vi "ClsGetNextMultipleSamplesSingleChannelDevice.vi"(7 "Time out(ms)":i32, 8 "error in (no error)":errorcluster, 10 "Number of Samples":i32, 11 "Connection In":u32) -> (0 "error out":errorcluster, 1 "If Timeout?":bool, 2 "_Data":dbl[][](array[numeric]), 3 "Connection Out":u32)   [LabVIEW 2010]
doc: "Get Next Multiple Samples:\n\nThis function is used for single channel devices. This function is used to get the next multiple valid samples from device. Use this function to avoid the overheads for having to call Get Next Sample subVI once to read each sample. It is especially useful when the data rate is high. This function is block but with timeout input available.\n\nConnection In[Input]: the connection handle which is initially created by Open Connection subVI.\n\nTimeout(milisecond)[Input]: in miliseconds, the subvi will return after the timeout no matter enough data are read or not. If set to -1, the timeout will be infinity and it will block until enough data are read.\n\nNumber of Samples[Input]: the number of samples to read for each call. The maximum of this number is only determined by the available memory of your PC.\n\n\nData[Output]: The two dimensional array for data. Note that you can use Get Signal IDs subVI to see the ordering of signal IDs correspondent to this data array. The first dimension is for different samples and the second dimension is for different signals. The number of samples may be less than expected if timeout.\n\nTimeout?[Output]: Whether the return of the function is a result of timeout.\n\nConnection Out[Output]: the connection handle output which could be used for next subVI refering to the same connection."
uses:
  tmp/CHRocodile VIS 1.1/dependent dlls/CHRocodileDLL.dll
panel:
  out "Number of data points":i32
  out "Singal IDs":i32[](array[numeric])
  out "Number of signals":i32
  out "initialized array":dbl[][](array[numeric])
  out "sucessful size check?":i32
  out "number of loops with check":i32
  out "Nr of Samples Returned":i32
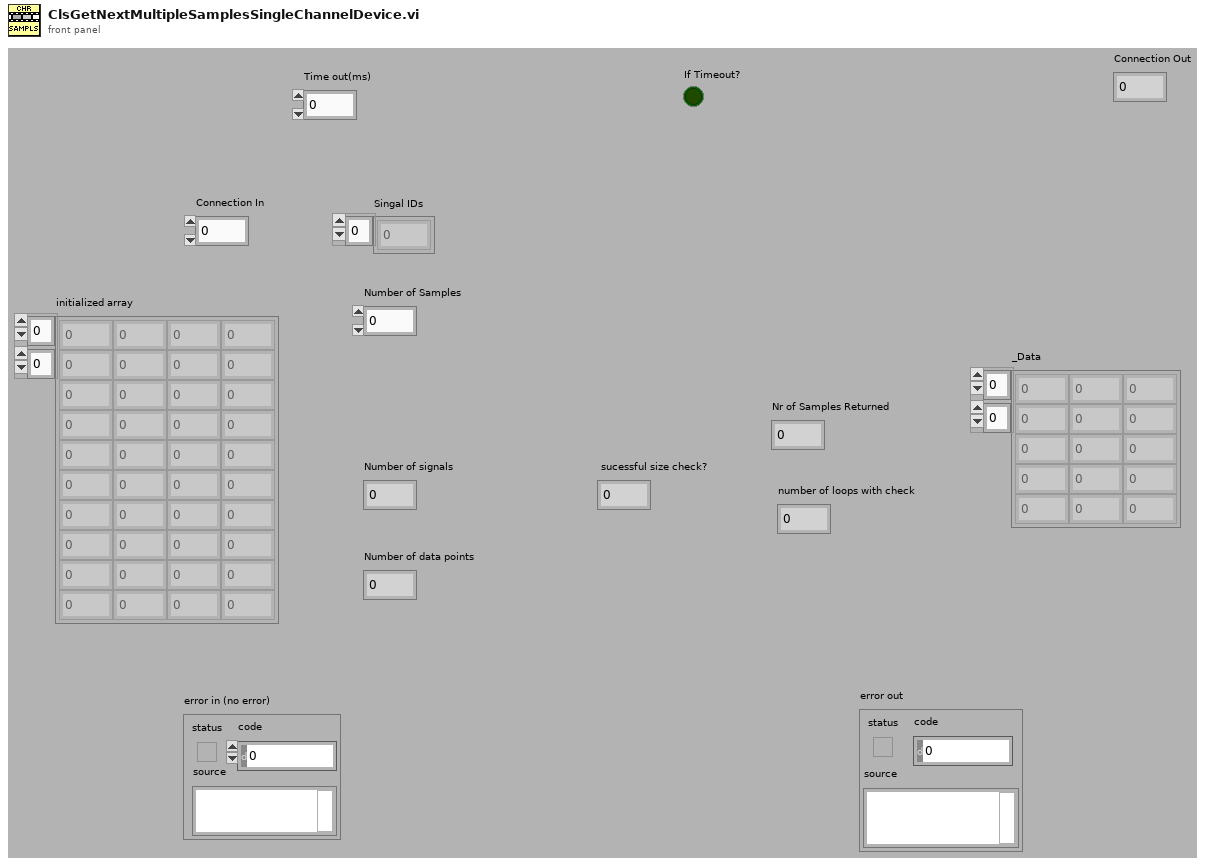
[diagram p1: front panel]
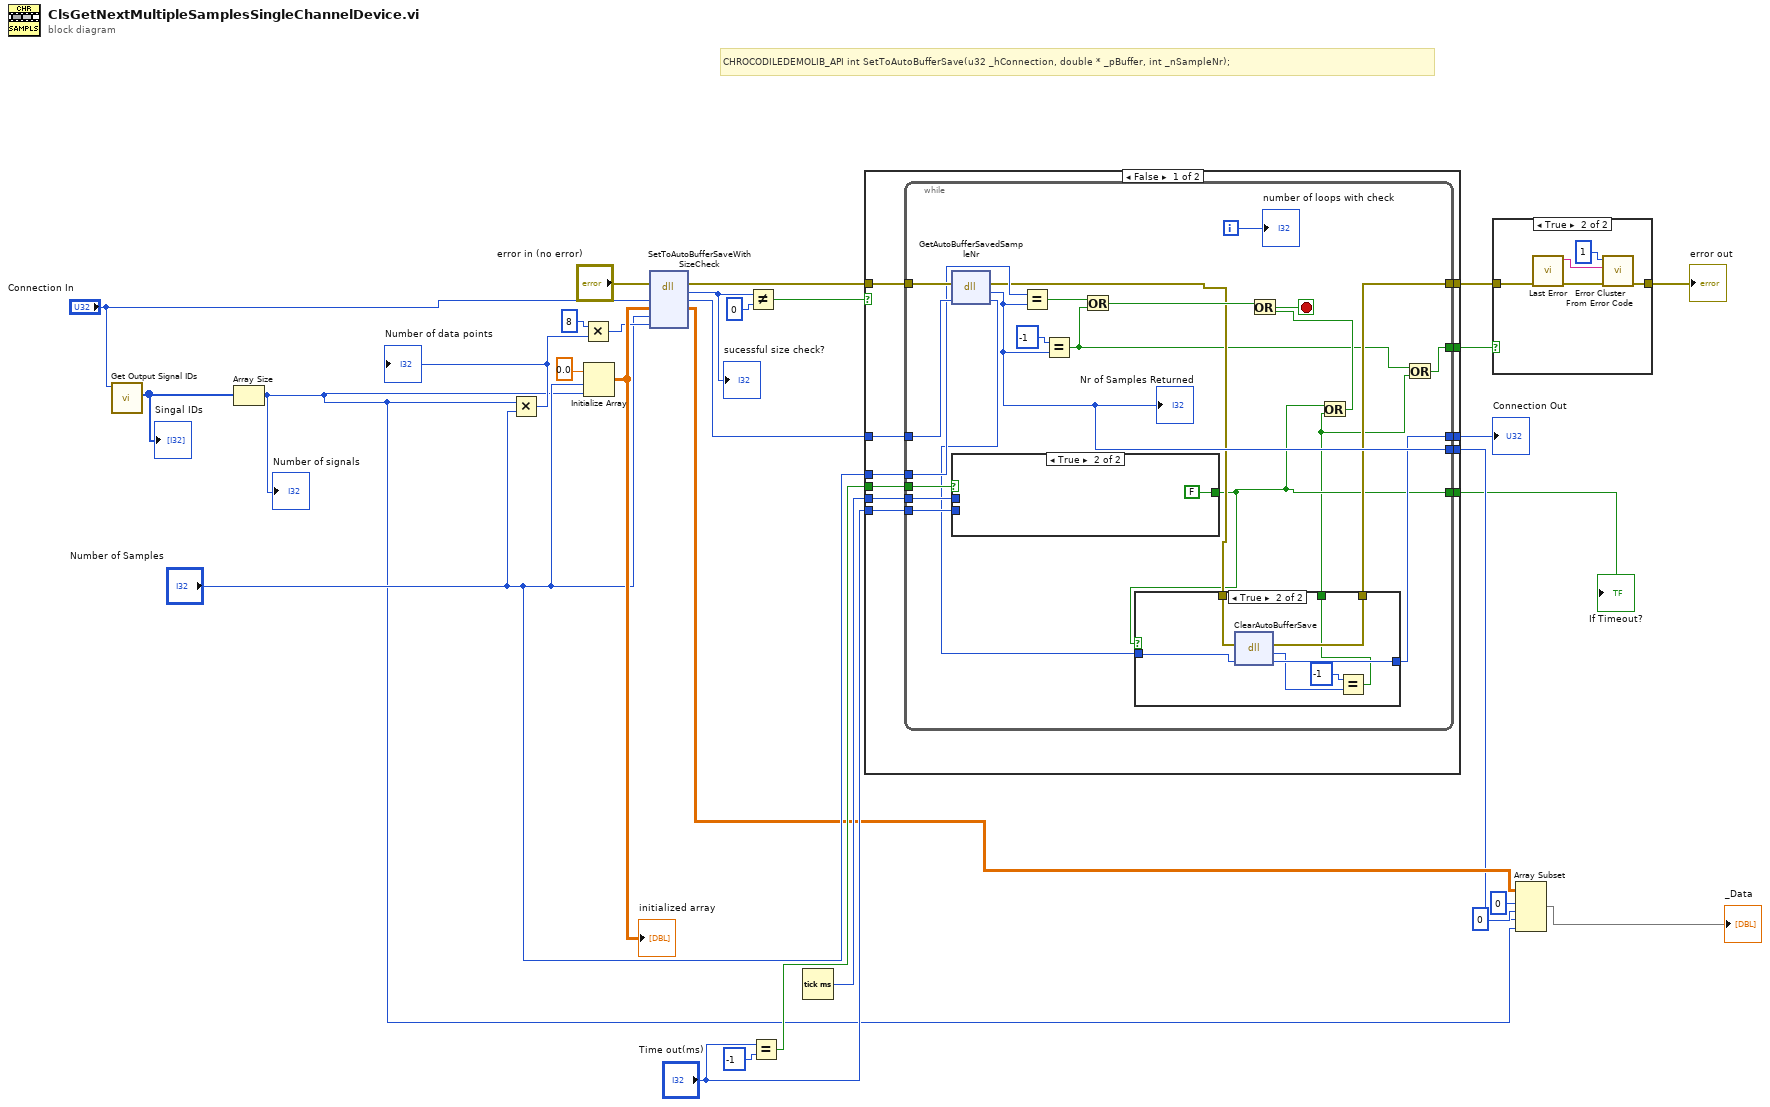
[diagram p0: block diagram]
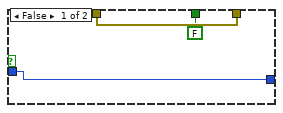
[diagram p2: hidden frame]
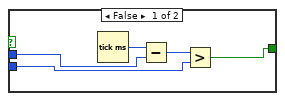
[diagram p3: hidden frame]
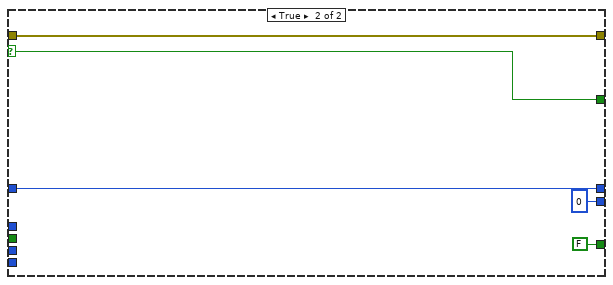
[diagram p4: hidden frame]
diagram:
  # "CHROCODILEDEMOLIB_API int SetToAutoBufferSave(u32 _hConnection, double * _pBuffer, int _nSampleNr);"
  n1 = call "Get Output Signal IDs.vi"("Connection In"="Connection In") -> ("Singal IDs"=w23:i32[])  [unwired: 8 in, 2 out]
  "Singal IDs" <- w23
  n2 = Array Size(array=w23) -> (size(s)=w4:i32)
  "Number of signals" <- w4
  n3 = Multiply(x=w4, y="Number of Samples") -> (x*y=w19:i32)
  "Number of data points" <- w19
  n4 = Multiply(x=8, y=w19) -> (x*y=w21:i32)
  n5 = Initialize Array(0.0 ("element"), "Number of Samples", w4) -> (w27:dbl[][])
  "initialized array" <- w27
  n6 = dll-call lib="C:/Users/y.ji/Desktop/tmp/CHRocodile VIS 1.1/dependent dlls/CHRocodileDLL.*" fn="SetToAutoBufferSaveWithSizeCheck"(error in="error in (no error)", "_hConnection"="Connection In", "_pBuffer"=w27, "_nSampleNr"="Number of Samples", "_pSizeCheck"=w21) -> (error out=w25:errorcluster, "return type"=w18:i32, "_hConnection"=w20:u32, "_pBuffer"=w7:dbl[][])  [unwired: 4 in, 1 out]
  "sucessful size check?" <- w18
  n7 = Not Equal?(x=w18, y=0) -> (x != y?=w16:bool)
  n8 = Equal?(x="Time out(ms)", y=-1) -> (x = y?=w12:bool)
  n9 = Tick Count (ms)() -> (millisecond timer value=w14:u32)
  n10 = case shown="False" w16 {
    selector: w16 -> [_ w80]
    tunnel: [w40 w82] -> w28
    tunnel: w25 -> [w39 w82]
    tunnel: w20 -> [w38 w81]
    tunnel: "Number of Samples" -> [w37 _]
    tunnel: [w32 w81] -> w10
    tunnel: [w36 w80] -> w15
    tunnel: w14 -> [w35 _]
    tunnel: w12 -> [w34 _]
    tunnel: "Time out(ms)" -> [w33 _]
    tunnel: [w31 0 ("return type")] -> w5
    tunnel: [w30 FALSE] -> w1
    frame False {
      n11 = while {
        tunnel: [w48] -> w40
        tunnel: w39 -> [w60]
        tunnel: w38 -> [w61]
        tunnel: [w46] -> w32
        tunnel: w37 -> [w59]
        tunnel: [w41] -> w36
        tunnel: w35 -> [w56]
        tunnel: w34 -> [w55]
        tunnel: w33 -> [w54]
        tunnel: [w50] -> w31
        tunnel: [w45] -> w30
        i -> [w51]
        stop <- w52 stop-if-true
        n12 = dll-call lib="C:/Users/y.ji/Desktop/tmp/CHRocodile VIS 1.1/dependent dlls/CHRocodileDLL.*" fn="GetAutoBufferSavedSampleNr"(error in=w60, "_hConnection"=w61) -> (error out=w49:errorcluster, "return type"=w50:i32, "_hConnection"=w47:u32)  [unwired: 2 in, 1 out]
        "Nr of Samples Returned" <- w50
        n13 = case shown="True" w55 {
          tunnel: w56 -> [w76 _]
          tunnel: w54 -> [w74 _]
          tunnel: [w72 FALSE] -> w45
          frame False {
            n14 = Tick Count (ms)() -> (millisecond timer value=w73:u32)
            n15 = Subtract(x=w73, y=w76) -> (x-y=w75:u32)
            n16 = Greater?(x=w75, y=w74) -> (0:w72:bool)
          }
          frame True {
          }
        }
        n17 = Equal?(x=w59, y=w50) -> (x = y?=w57:bool)
        n18 = Equal?(x=-1, y=w50) -> (x = y?=w43:bool)
        n19 = Or(x=w57, y=w43) -> (x .or. y?=w53:bool)
        n20 = case shown="True" w45 {
          tunnel: w49 -> [w64 w71]
          tunnel: [w64 w70] -> w48
          tunnel: w47 -> [w63 w69]
          tunnel: [w63 w68] -> w46
          tunnel: [FALSE w65] -> w42
          frame False {
          }
          frame True {
            n21 = dll-call lib="C:/Users/y.ji/Desktop/tmp/CHRocodile VIS 1.1/dependent dlls/CHRocodileDLL.*" fn="ClearAutoBufferSave"(error in=w71, "_hConnection"=w69) -> (error out=w70:errorcluster, "return type"=w66:i32, "_hConnection"=w68:u32)  [unwired: 2 in, 1 out]
            n22 = Equal?(x=-1, y=w66) -> (x = y?=w65:bool)
          }
        }
        n23 = Or(x=w45, y=w42) -> (x .or. y?=w44:bool)
        n24 = Or(x=w53, y=w44) -> (x .or. y?=w52:bool)
        n25 = Or(x=w43, y=w42) -> (x .or. y?=w41:bool)
        "number of loops with check" <- w51
      }
    }
    frame True {
    }
  }
  "Connection Out" <- w10
  "If Timeout?" <- w1
  n26 = case shown="True" w15 {
    tunnel: [w83 w87] -> w29
    tunnel: w28 -> [w83 w84]
    frame False {
    }
    frame True {
      n27 = call "Last Error.vi"("error in (no error)"=w84) -> ("error out"=w85:errorcluster, "Error Message"=w86:string)  [unwired: 9 in]
      n28 = call <vilib>:"Error Cluster From Error Code.vi"("error in (no error)"=w85, "error message (\"\")"=w86, "error code (0)"=1) -> ("error out"=w87:errorcluster)  [unwired: 6 in]
    }
  }
  "error out" <- w29
  n29 = Array Subset(array=w7, index (row)=0 ("index"), length (row)=w5, index (col)=0 ("index"), length (col)=w4) -> (→"_Data":dbl[][])
